vi "Acoustic Frequency Response Stepped Sine Sweep.vi"(0 "TSM context":T2, 5 "Freq Sweep":T1={"Start"=1.0, "End"=10.0, "Samples"=128} {"End" format="%#_13g"; "Start" format="%#_13g"}, 11 "dB SPL":dbl=1000.0, 12 "Duration":dbl=2.0 format="%#_6p", 13 "Duration in Cycles? (F)":bool) -> (15 "error out":errorcluster)   [LabVIEW 2020]
doc: "Acoustic THD Response measure the THD of the DUT at various acoustic stimuli (dB SPL) with constant frequency and duration. Acoustic Functional Response Stepped Sine is used to get the THD (%) of the DUT."
uses:
  <vilib>/NI_TestStand_SemiconductorModule/NI_TestStand_Semiconductor_Module.lvlibp/PinMap/General/SemiconductorModuleContext.ctl
  Common/Utility/Calibration Sweep/Sweep Parameters.ctl
  Typedefs/Acoustic Sweep Config Cluster.ctl
  <vilib>/Analysis/1siggen.llb/Ramp Pattern.vi
  <vilib>/Analysis/1siggen.llb/Ramp Pattern by Samples.vi
  <vilib>/Utility/error.llb/Error Cluster From Error Code.vi
  <vilib>/NI_TestStand_SemiconductorModule/NI_TestStand_Semiconductor_Module.lvlibp
panel:
  out "Frequency Response":cluster{"X":dbl, "Y":dbl}[](graph)
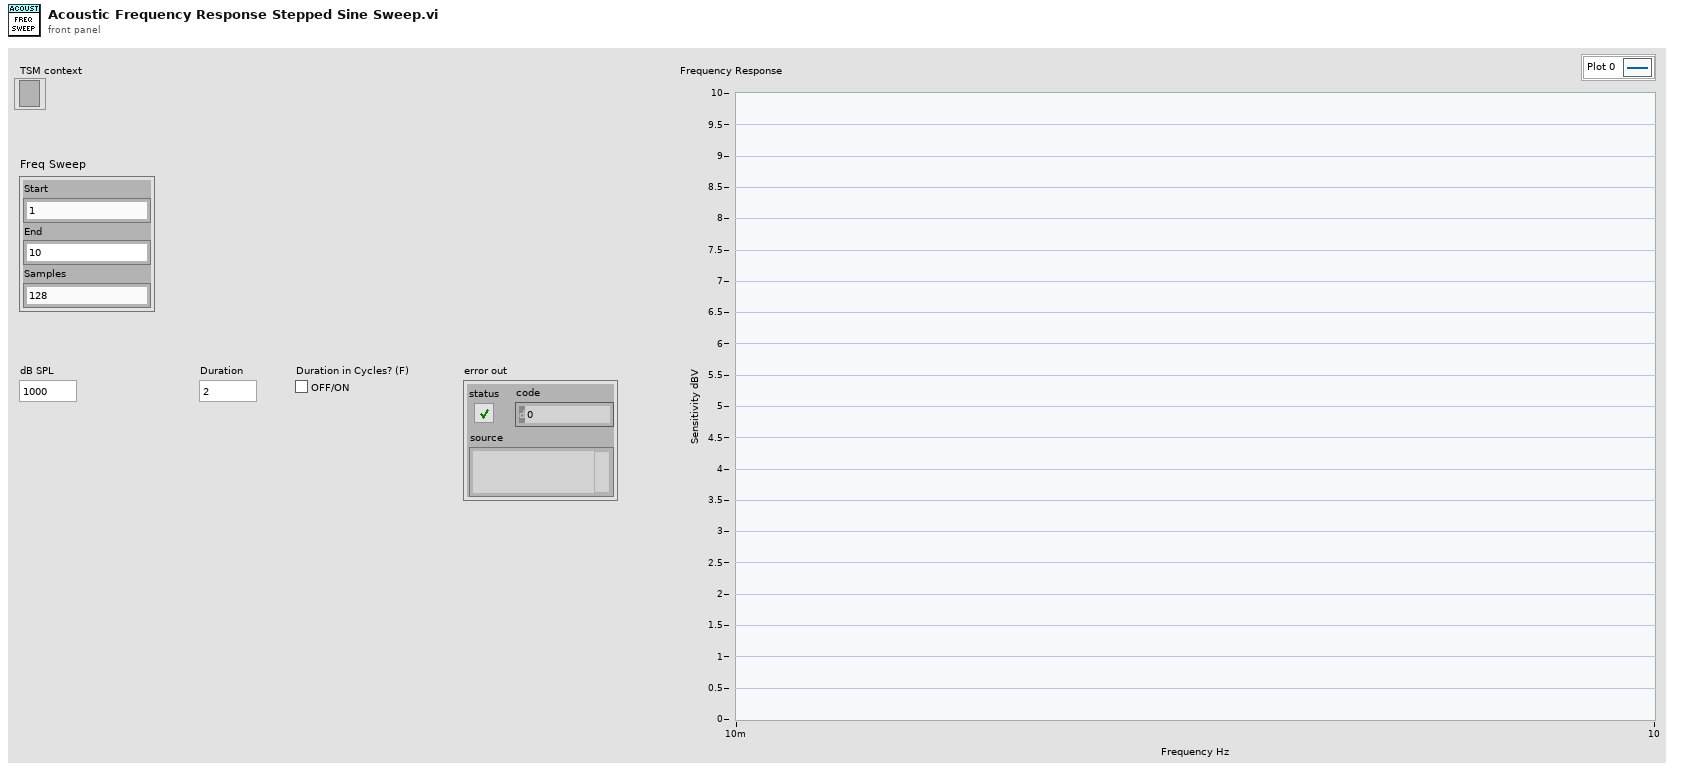
[diagram p1: front panel]
types:
  T1 = typedef "Sweep Parameters.ctl" = cluster{"Start":dbl, "End":dbl, "Samples":i32}
  T2 = typedef "NI_TestStand_Semiconductor_Module.lvlibp/SemiconductorModuleContext.ctl" = refnum<k7>
  T3 = typedef "Acoustic Sweep Config Cluster.ctl" = cluster{"Frequency":dbl, "dB SPL":dbl, "Duration":dbl}
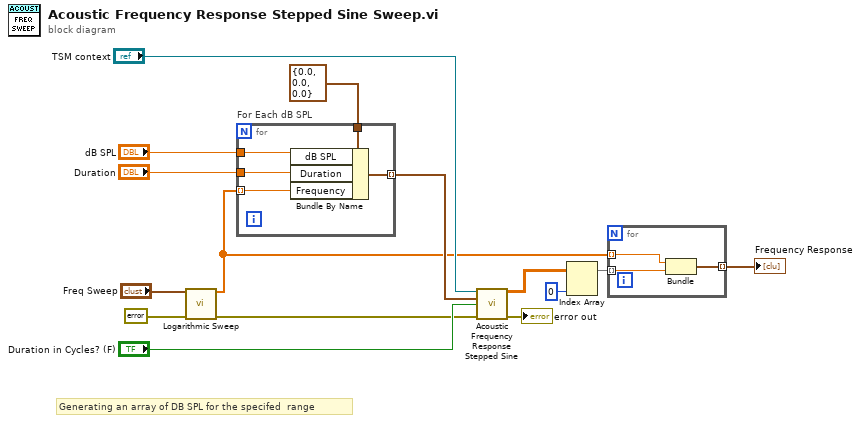
[diagram p0: block diagram]
diagram:
  # "Generating an array of DB SPL for the specifed  range"
  n1 = call "Logarithmic Sweep.vi"("Sweep Parameters"="Freq Sweep", "error in (no error)"=errorcluster {"status"=FALSE, "code"=0, "source"=""}) -> ("Ramp Pattern"=w2:dbl[], "error out"=w9:errorcluster)  [unwired: 12 in]
  n2 = for "For Each dB SPL" {
    tunnel: T3 {"Frequency"=0.0, "dB SPL"=0.0, "Duration"=0.0} ("Cluster") -> [w20]
    tunnel: w2 -> [w16] mode=indexing
    tunnel: "Duration" -> [w19]
    tunnel: "dB SPL" -> [w18]
    tunnel: [w17] -> w14 mode=indexing
    n3 = Bundle By Name(cluster=w20, "dB SPL"=w18, "Duration"=w19, "Frequency"=w16) -> (w17:T3)
  }
  n4 = call "Acoustic Frequency Response Stepped Sine.vi"("TSM context"="TSM context", "Sweep Configuration"=w14, "Duration in Cycles? (F)"="Duration in Cycles? (F)", "error in (no error)"=w9) -> ("DUT Measurements"=w5:dbl[][], "error out"=→"error out":errorcluster)  [unwired: 9 in, 1 out]
  n5 = Index Array(array=w5, index (col)=0 ("disabled index (col)")) -> (element=w4:dbl[])  [unwired: 1 in]
  n6 = for {
    tunnel: w4 -> [w23] mode=indexing
    tunnel: w2 -> [w22] mode=indexing
    tunnel: [w21] -> w1 mode=indexing
    n7 = Bundle(w22, "THD"=w23) -> (w21:cluster{dbl, "THD":dbl})  [unwired: 1 in]
  }
  "Frequency Response" <- w1
